vi "mixer.vi"(1 "参考信号":dbl[](array[numeric]), 2 "中频信号":dbl[](array[numeric])) -> (0 "混频信号输出":dbl[](array[numeric]))   [LabVIEW 2018]
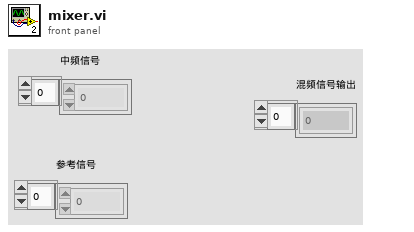
[diagram p1: front panel]
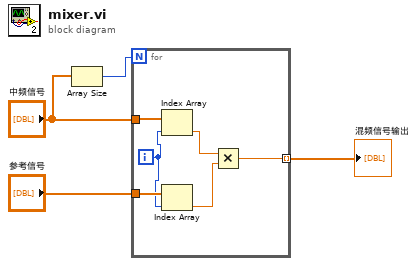
[diagram p0: block diagram]
diagram:
  n1 = Array Size(array="中频信号") -> (size(s)=w4:i32)
  n2 = for {
    N: w4 -> [_]
    tunnel: "中频信号" -> [w10]
    tunnel: "参考信号" -> [w9]
    tunnel: [w5] -> w1 mode=indexing
    i -> [w8]
    n3 = Index Array(array=w10, index=w8) -> (element=w7:dbl)
    n4 = Index Array(array=w9, index=w8) -> (element=w6:dbl)
    n5 = Multiply(x=w7, y=w6) -> (x*y=w5:dbl)
  }
  "混频信号输出" <- w1
